vi "Decorator.vi"(10 "Actor":refnum<class "Actor.lvclass">, 11 "jettl Actor in":refnum<class "jettl Actor.lvclass">) -> (3 "jettl Actor out":refnum<class "jettl Actor.lvclass">)   [LabVIEW 2021, in "jettl.lvlib" / "Temporary Actor.lvlib" / "jettl Actor.lvclass"]
uses:
  jettl Actor.lvclass
  Actor/Actor.lvclass
  jettl Actor.lvclass/jettl Actor.ctl
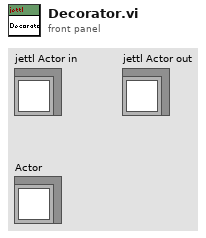
[diagram p1: front panel]
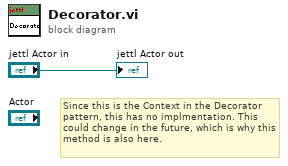
[diagram p0: block diagram]
diagram:
  # "Since this is the Context in the Decorator pattern, this has no implmentation. This could change in the future, which is why this method is also here."
  "jettl Actor out" <- "jettl Actor in"
